vi "ReadAOs.vi"(8 "error in":errorcluster, 10 "Analog Output":T2, 11 "VISA resource name":refnum<visa-resource-name>) -> (0 "error out":errorcluster, 2 "AnOutValues":T1 {"Frequency" format="%#pHz"; "Duty" format="%.02f%%"}, 3 "VISA resource name out":refnum<visa-resource-name>)   [LabVIEW 2020, in "HandsOnPi2040.lvlib"]
uses:
  HandsOnPi2040.lvlib
  AOs.ctl
  PWMSettings.ctl
  <vilib>/CTI/CTI Visa Drivers/CTI-Visa/CTI-Visa.lvlib
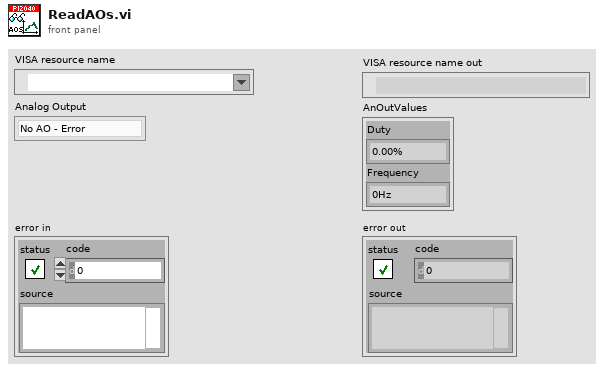
[diagram p1: front panel]
types:
  T1 = typedef "HandsOnPi2040.lvlib/PWMSettings.ctl" = cluster{"Duty":sgl, "Frequency":sgl}
  T2 = typedef "HandsOnPi2040.lvlib/AOs.ctl" = enum8{"No AO - Error", "AO1 (GPIO28)"}
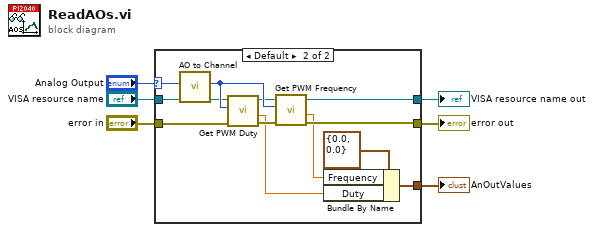
[diagram p0: block diagram]
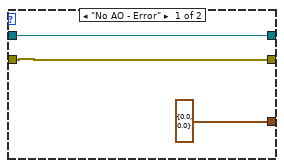
[diagram p2: hidden frame]
diagram:
  n1 = case shown="Default" "Analog Output" {
    selector: "Analog Output" -> [_ w10]
    tunnel: "VISA resource name" -> [w8 w17]
    tunnel: "error in" -> [w9 w20]
    tunnel: [w8 w14] -> w4
    tunnel: [w9 w18] -> w5
    tunnel: [T1 {"Duty"=0.0, "Frequency"=0.0} ("AnOutValues") w11] -> w1
    frame "No AO - Error" {
    }
    frame Default {
      n2 = call "AO to Channel.vi"("Analog Output"=w10) -> ("Channel"=w21:i32)  [unwired: 10 in]
      n3 = call <vilib>:"Get PWM Duty.vi"("error in (no error)"=w20, "Channel"=w21, "VISA resource name in"=w17) -> ("error out"=w19:errorcluster, "Duty % (0-1)"=w12:sgl, "VISA resource name"=w15:refnum<visa-resource-name>)  [unwired: 6 in]
      n4 = call <vilib>:"Get PWM Frequency.vi"("error in (no error)"=w19, "Channel"=w21, "VISA resource name in"=w15) -> ("error out"=w18:errorcluster, "Freq Hz"=w13:sgl, "VISA resource name"=w14:refnum<visa-resource-name>)  [unwired: 6 in]
      n5 = Bundle By Name(cluster=T1 {"Duty"=0.0, "Frequency"=0.0} ("AnOutValues"), "Frequency"=w13, "Duty"=w12) -> (w11:T1)
    }
  }
  "VISA resource name out" <- w4
  "AnOutValues" <- w1
  "error out" <- w5
